vi "Gas_Remaining.vi"() -> (0 "Kg Remaining":dbl[](array[numeric]) format="%.9f", 1 "Gas names":string[](array[string]))   [LabVIEW 2020]
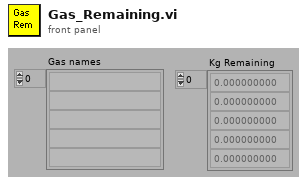
[diagram p1: front panel]
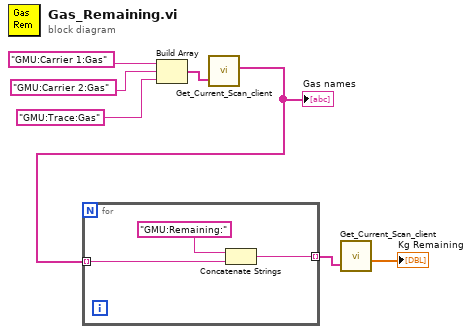
[diagram p0: block diagram]
diagram:
  n1 = Build Array("GMU:Carrier 1:Gas", "GMU:Carrier 2:Gas", "GMU:Trace:Gas") -> (w4:string[])
  n2 = call "Get_Current_Scan_client.vi"("multipleChannels"=w4) -> ("String values"=w6:string[])  [unwired: 2 in, 2 out]
  "Gas names" <- w6
  n3 = for {
    tunnel: w6 -> [w9] mode=indexing
    tunnel: [w8] -> w7 mode=indexing
    n4 = Concatenate Strings("GMU:Remaining:", w9) -> (w8:string)
  }
  n5 = call "Get_Current_Scan_client.vi"("multipleChannels"=w7) -> ("Numerical Values"=→"Kg Remaining":dbl[])  [unwired: 2 in, 2 out]
